vi "String to char Array.vi"(11 "Row":string) -> (3 "Array":string[](array[string]))   [LabVIEW 2021, in "Helpers.lvlib"]
uses:
  Day 12/Proto/Group.lvclass/Group.ctl
  Helpers.lvlib
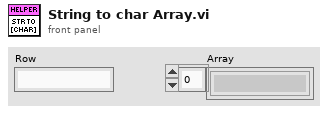
[diagram p1: front panel]
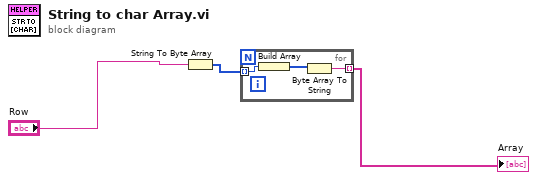
[diagram p0: block diagram]
diagram:
  n1 = String To Byte Array(string="Row") -> (unsigned byte array=w1:u8[])
  n2 = for {
    tunnel: w1 -> [w6] mode=indexing
    tunnel: [w4] -> w3 mode=indexing
    n3 = Build Array(w6) -> (w5:u8[])
    n4 = Byte Array To String(unsigned byte array=w5) -> (string=w4:string)
  }
  "Array" <- w3
